vi "RS232_Hook.vi"(0 "RS232 Config":T2={"VISA resource name"="COM1", "baud rate"=9600, "data bits"=8, "parity"=0, "stop bits"=10} {"stop bits" items=["1.0"=10, "1.5"=15, "2.0"=20]; "parity" items=["None", "Odd", "Even", "Mark", "Space"]; "data bits" min=5 max=8 step=1}, 2 "Mode":T1(ring), 7 "data in":string, 11 "error in":errorcluster) -> (6 "data out":string, 15 "error out":errorcluster)   [LabVIEW 2011]
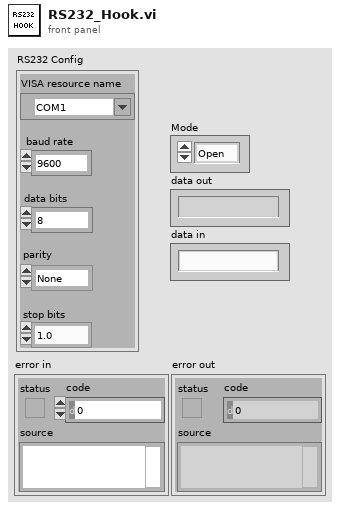
[diagram p1: front panel]
types:
  T1 = enum16{"Open", "R", "W", "R->W", "W->R", "Close"}
  T2 = cluster{"VISA resource name":refnum<visa-resource-name>, "baud rate":u32, "data bits":u16, "parity":u16, "stop bits":u16}
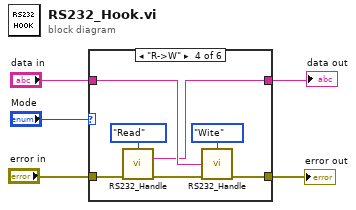
[diagram p0: block diagram]
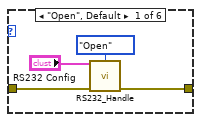
[diagram p2: hidden frame]
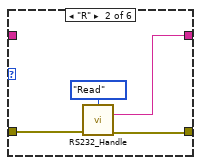
[diagram p3: hidden frame]
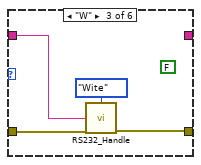
[diagram p4: hidden frame]
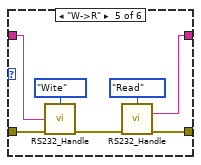
[diagram p5: hidden frame]
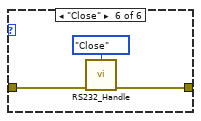
[diagram p6: hidden frame]
diagram:
  n1 = case shown="\"R->W\"" "Mode" {
    tunnel: "error in" -> [w9 w13 w17 w24 w28 w34]
    tunnel: [w8 w12 w16 w22 w27 w33] -> w4
    tunnel: "data in" -> [_ _ w14 w19 w26 _]
    tunnel: [_ w10 _ w18 w25 _] -> w2
    frame "Open", Default {
      n2 = call "RS232_Handle.vi"("Config"="RS232 Config", "Handle"=enum16{"Open", "Read", "Wite", "Close"}."Open", "error in"=w9) -> ("error out"=w8:errorcluster)  [unwired: 11 in, 1 out]
    }
    frame "R" {
      n3 = call "RS232_Handle.vi"("Handle"=enum16{"Open", "Read", "Wite", "Close"}."Read", "error in"=w13) -> ("data out"=w10:string, "error out"=w12:errorcluster)  [unwired: 12 in]
    }
    frame "W" {
      (unwired) FALSE ("ok")
      n4 = call "RS232_Handle.vi"("Handle"=enum16{"Open", "Read", "Wite", "Close"}."Wite", "data in"=w14, "error in"=w17) -> ("error out"=w16:errorcluster)  [unwired: 11 in, 1 out]
    }
    frame "R->W" {
      n5 = call "RS232_Handle.vi"("Handle"=enum16{"Open", "Read", "Wite", "Close"}."Read", "error in"=w24) -> ("data out"=w18:string, "error out"=w23:errorcluster)  [unwired: 12 in]
      n6 = call "RS232_Handle.vi"("Handle"=enum16{"Open", "Read", "Wite", "Close"}."Wite", "data in"=w19, "error in"=w23) -> ("error out"=w22:errorcluster)  [unwired: 11 in, 1 out]
    }
    frame "W->R" {
      n7 = call "RS232_Handle.vi"("Handle"=enum16{"Open", "Read", "Wite", "Close"}."Wite", "data in"=w26, "error in"=w28) -> ("error out"=w31:errorcluster)  [unwired: 11 in, 1 out]
      n8 = call "RS232_Handle.vi"("Handle"=enum16{"Open", "Read", "Wite", "Close"}."Read", "error in"=w31) -> ("data out"=w25:string, "error out"=w27:errorcluster)  [unwired: 12 in]
    }
    frame "Close" {
      n9 = call "RS232_Handle.vi"("Handle"=enum16{"Open", "Read", "Wite", "Close"}."Close", "error in"=w34) -> ("error out"=w33:errorcluster)  [unwired: 12 in, 1 out]
    }
  }
  "error out" <- w4
  "data out" <- w2
